vi "Time Stamp to Data Type.vi"(8 "error in (no error)":errorcluster, 11 "Time Stamp":timestamp) -> (0 "error out":errorcluster, 3 "Boolean out":refnum<class "Timestamp.lvclass">)   [LabVIEW 2017, in "Timestamp.lvclass"]
uses:
  <vilib>/gpm_packages/@cs/data-type-serializer/source/Timestamp/Timestamp.lvclass
  <vilib>/gpm_packages/@cs/data-type-serializer/source/Timestamp/Timestamp.lvclass/Timestamp.ctl
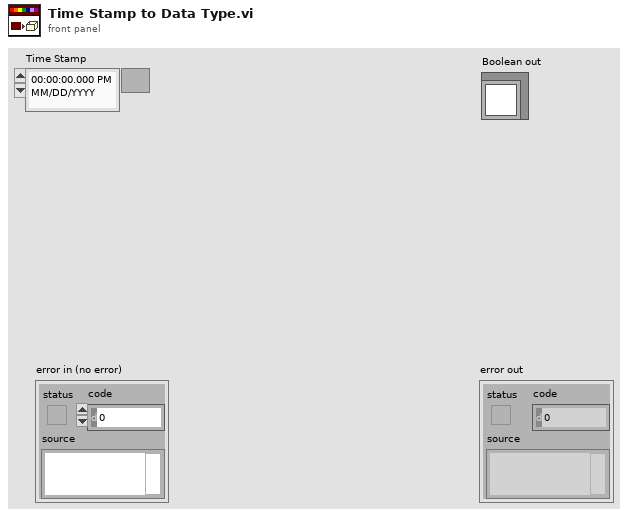
[diagram p1: front panel]
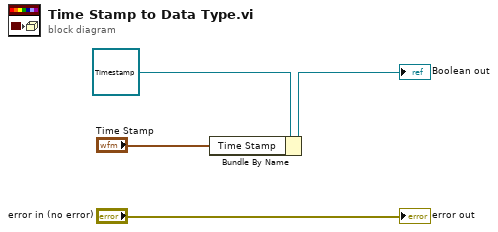
[diagram p0: block diagram]
diagram:
  n1 = Bundle By Name(cluster=refnum<class "Timestamp.lvclass"> refnum ("Boolean in"), "Time Stamp"="Time Stamp") -> (→"Boolean out":refnum<class "Timestamp.lvclass">)
  "error out" <- "error in (no error)"
